vi "testAppendErrorInformation_NoError_withoutState.vi"(8 "error in (no error)":errorcluster, 11 "testStateMachineUtilities in":refnum<class "testStateMachineUtilities.lvclass">) -> (0 "error out":errorcluster, 3 "testStateMachineUtilities out":refnum<class "testStateMachineUtilities.lvclass">)   [LabVIEW 2013, in "testStateMachineUtilities.lvclass"]
uses:
  testStateMachineUtilities.lvclass
  source/State Machine Support API/Parse State Queue_2024.vi
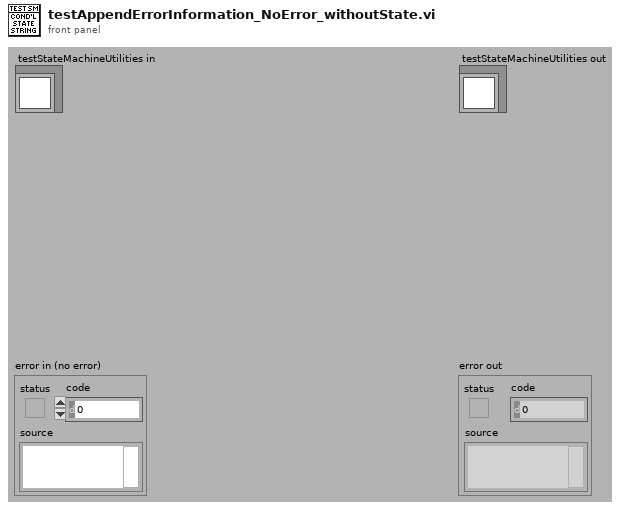
[diagram p1: front panel]
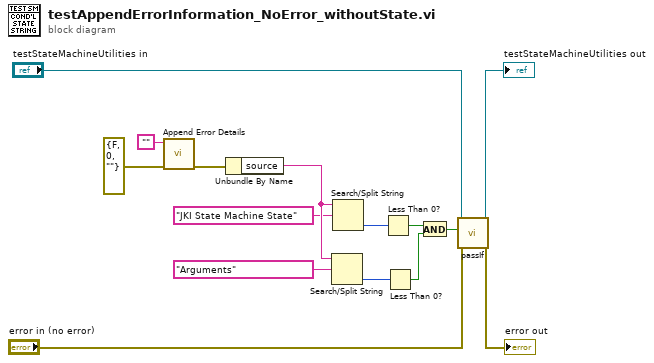
[diagram p0: block diagram]
diagram:
  n1 = call "Append Error Details.vi"("error in (no error)"=errorcluster {"status"=FALSE, "code"=0, "source"=""}, "Previous State and Argument(s)"="") -> ("error out"=w6:errorcluster)  [unwired: 9 in]
  n2 = Unbundle By Name(w6) -> ("source"=w5:string)
  n3 = Search/Split String(string=w5, search string/char (-)="Arguments") -> (offset of match=w10:i32)  [unwired: 1 in, 2 out]
  n4 = Search/Split String(string=w5, search string/char (-)="JKI State Machine State") -> (offset of match=w11:i32)  [unwired: 1 in, 2 out]
  n5 = Less Than 0?(x=w11) -> (x < 0?=w9:bool)
  n6 = Less Than 0?(x=w10) -> (x < 0?=w8:bool)
  n7 = And(x=w9, y=w8) -> (x .and. y?=w7:bool)
  n8 = call-dynamic "passIf.vi"("error in (no error)"="error in (no error)", "pass"=w7, "TestCase in"="testStateMachineUtilities in") -> ("error out"=→"error out":errorcluster, "TestCase out"=→"testStateMachineUtilities out":refnum<class "testStateMachineUtilities.lvclass">)  [unwired: 7 in]
